vi "TDCObj to hit.vi"(8 "error in":errorcluster, 10 "TDCHits Buffer":T1, 11 "#of hits":i32) -> (0 "error out":errorcluster, 1 "Array":T2[](array[typedef]))   [LabVIEW 2016, in "HPTDC Driver Library.lvlib"]
uses:
  HPTDC Driver Library.lvlib
  Typedefs/TDCHit.ctl
  Typedefs/TDCHitObjBuffer.ctl
  C:/Users/CRT Controller/CRTC Labview Application/Source/HPTDC Driver Library Folder/Library files/hptdc_net4_3.7.0_x64.dll
  hptdc_net4_3.7.0_x64.dll
  VIs/Global Variables/Global Resolution.vi
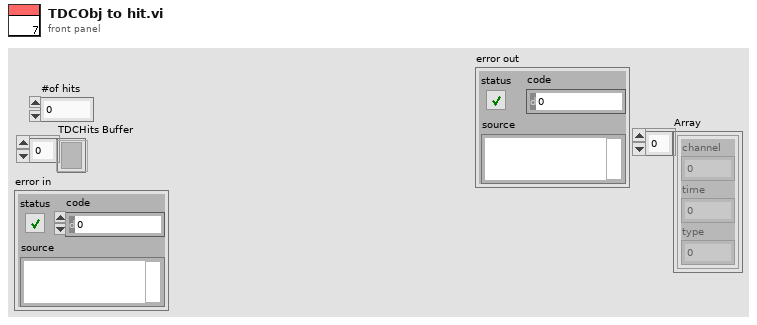
[diagram p1: front panel]
types:
  T1 = typedef "TDCHitObjBuffer.ctl" = refnum<k24>[]
  T2 = typedef "HPTDC Driver Library.lvlib/TDCHit.ctl" = cluster{"channel":u8, "time":u64, "type":u8}
  T3 = enum16{"insertPPS", "insertUTC", "read", "initiate"}
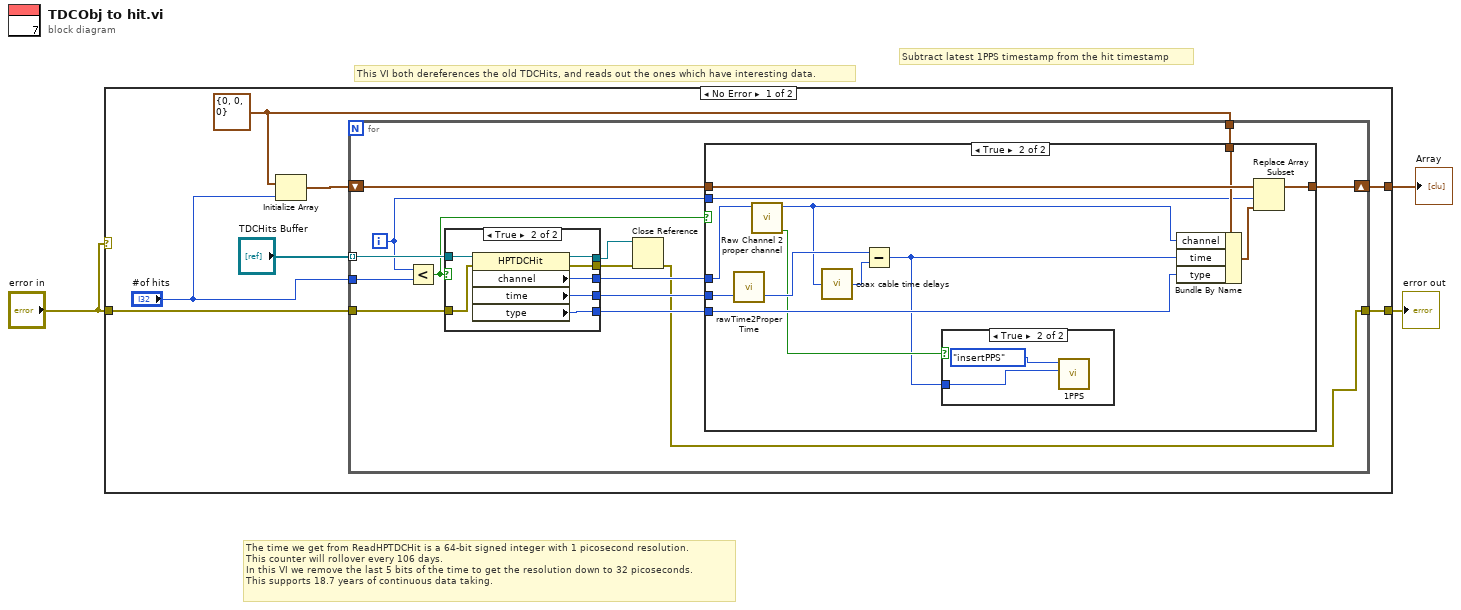
[diagram p0: block diagram]
diagram:
  # "Subtract latest 1PPS timestamp from the hit timestamp"
  # "This VI both dereferences the old TDCHits, and reads out the ones which have interesting data."
  # "The time we get from ReadHPTDCHit is a 64-bit signed integer with 1 picosecond resolution.\nThis counter will rollover every 106 days.\nIn this VI we remove the last 5 bits of the time to get the resolution down to 32 picoseconds.\nThis supports 18.7 years of continuous data taking."
  n1 = case shown="No Error" "error in" {
    tunnel: [w8 _] -> w3
    tunnel: "error in" -> [w5 w50]
    tunnel: [w4 w50] -> w2
    frame No Error {
      w7 = T2 {"channel"=0, "time"=0, "type"=0} ("element")
      n2 = Initialize Array(w7, "#of hits") -> (w9:T2[])
      n3 = for {
        tunnel: "TDCHits Buffer" -> [w24] mode=indexing
        shift-right: [w20] -> w8
        shift-left: w9 -> [w21]
        tunnel: w7 -> [w19]
        tunnel: "#of hits" -> [w13]
        tunnel: w5 -> [w15]
        tunnel: [w11] -> w4
        i -> [w14]
        n4 = Less?(x=w14, y=w13) -> (x < y?=w17:bool)
        n5 = case shown="True" w17 {
          tunnel: w24 -> [w42 w43]
          tunnel: [_ w49] -> w23
          tunnel: [_ w48] -> w22
          tunnel: [w42 w47] -> w18
          tunnel: [w41 w46] -> w16
          tunnel: w15 -> [w41 w45]
          tunnel: [_ w44] -> w12
          frame False {
          }
          frame True {
            n6 = property class="HPTDCHit"(reference=w43, error in=w45) -> (reference out=w47:refnum<k24>, error out=w46:errorcluster, "channel"=w49:u8, "time"=w48:i64, "type"=w44:u8)
          }
        }
        n7 = Close Reference(reference=w18, error in (no error)=w16) -> (error out=w11:errorcluster)
        n8 = case shown="True" w17 {
          tunnel: w23 -> [_ w29]
          tunnel: w22 -> [_ w38]
          tunnel: w21 -> [w25 w37]
          tunnel: [w25 w36] -> w20
          tunnel: w19 -> [_ w34]
          tunnel: w14 -> [_ w33]
          tunnel: w12 -> [_ w31]
          frame False {
          }
          frame True {
            n9 = call "rawTime2ProperTime.vi"("Tdchhit time"=w38) -> ("32ps res unsigned"=w30:u64)  [unwired: 1 in, 1 out]
            n10 = call "Raw Channel 2 proper channel.vi"("channel in"=w29) -> ("PPS?"=w27:bool, "channel out"=w28:u8)  [unwired: 9 in]
            n11 = call "coax cable time delays.vi"("channel"=w28) -> ("Coax cable time (x32ps)"=w32:u64)
            n12 = Subtract(x=w30, y=w32) -> (x-y=w26:u64)
            n13 = case shown="True" w27 {
              tunnel: w26 -> [_ w40]
              frame False {
              }
              frame True {
                n14 = call "1PPS.vi"("1PPS ts"=w40, "Action"=T3."insertPPS") -> ()  [unwired: 2 in, 1 out]
              }
            }
            n15 = Bundle By Name(cluster=w34, "channel"=w28, "time"=w26, "type"=w31) -> (w35:T2)
            n16 = Replace Array Subset(array=w37, new element=w35, index=w33) -> (w36:T2[])
          }
        }
      }
    }
    frame Error {
    }
  }
  "Array" <- w3
  "error out" <- w2
